vi "check syntax_core.vi"(8 "error in (no error)":errorcluster caption="에러 입력(에러 없음)", 11 "Script Line_i2c sw 입력":refnum<class "Script Line_i2c sw.lvclass">) -> (0 "error out":errorcluster caption="에러 출력", 3 "Script Line_i2c sw 출력":refnum<class "Script Line_i2c sw.lvclass">)   [LabVIEW 2020, in "Script Line_i2c sw.lvclass"]
uses:
  Script Line_i2c sw.lvclass
  Script Line/Script Line.lvclass/Script Line.ctl
  Script Line_i2c/Script Line_i2c.lvclass/Script Line_i2c.ctl
  Script Line_i2c/Accessors/Write slv.vi
  Script Line_i2c/Accessors/Write reg.vi
  Script Line_i2c/Accessors/Write reg addr byte.vi
  Script Line_i2c/Accessors/Write size.vi
  Script Line_i2c/Accessors/Write data.vi
  Script Line/Accessors/Read parameter.vi
  Script Line/Accessors/Read parameter string index.vi
  Script Line/Script Line.lvclass
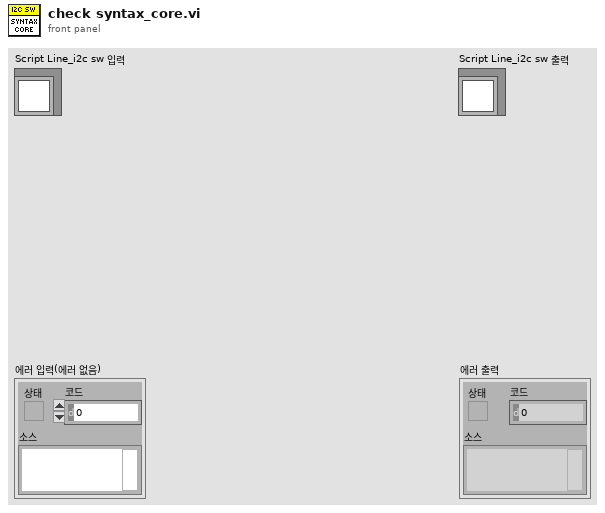
[diagram p1: front panel]
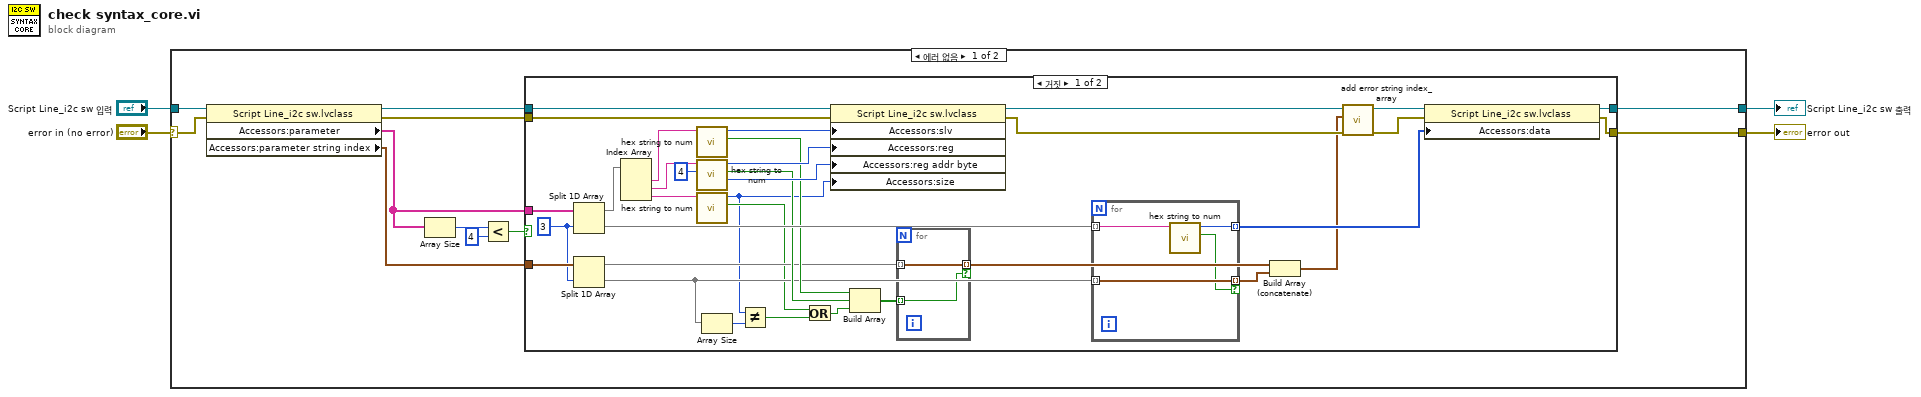
[diagram p0: block diagram]
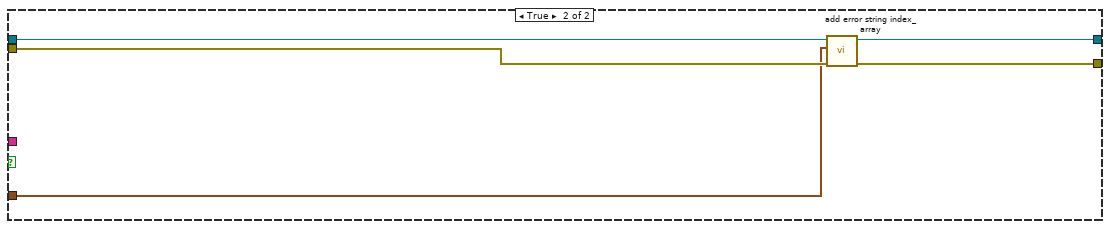
[diagram p2: hidden frame]
diagram:
  n1 = case shown="에러 없음" "error in (no error)" {
    selector: "error in (no error)" -> [w14 w62]
    tunnel: [w5 w62] -> w1
    tunnel: [w6 w61] -> w3
    tunnel: "Script Line_i2c sw 입력" -> [w15 w61]
    frame No Error {
      n2 = property class="Script Line_i2c sw.lvclass"(reference=w15, error in=w14) -> (reference out=w9:refnum<class "Script Line_i2c sw.lvclass">, error out=w8:errorcluster, "Accessors:parameter"=w10:string[], "Accessors:parameter string index"=w7:cluster{"start":u32, "end":u32}[])
      n3 = Array Size(array=w10) -> (size(s)=w13:i32)
      n4 = Less?(x=w13, y=4) -> (x < y?=w11:bool)
      n5 = case shown="거짓" w11 {
        tunnel: w10 -> [w49 _]
        tunnel: w7 -> [w48 w56]
        tunnel: w9 -> [w41 w58]
        tunnel: w8 -> [w42 w60]
        tunnel: [w45 w59] -> w5
        tunnel: [w43 w57] -> w6
        frame False {
          w37 = 3 ("길이")
          n6 = Split 1D Array(array=w49, index=w37) -> (first subarray=w36:string[], second subarray=w35:string[])
          n7 = Split 1D Array(array=w48, index=w37) -> (first subarray=w25:cluster{"start":u32, "end":u32}[], second subarray=w21:cluster{"start":u32, "end":u32}[])
          n8 = Index Array(array=w36) -> (element #1=w29:string, element #2=w30:string, element #3=w31:string)  [unwired: 3 in]
          n9 = call "hex string to num.vi"("string"=w29) -> ("error"=w27:bool, "num"=w32:u32)  [unwired: 7 in, 2 out]
          n10 = call "hex string to num.vi"("max byte (1)"=u8 4, "string"=w30) -> ("byte"=w39:u8, "error"=w26:bool, "num"=w40:u32)  [unwired: 6 in, 1 out]
          n11 = call "hex string to num.vi"("string"=w31) -> ("error"=w19:bool, "num"=w18:u32)  [unwired: 7 in, 2 out]
          n12 = Array Size(array=w21) -> (size(s)=w20:i32)
          n13 = Not Equal?(x=w18, y=w20) -> (x != y?=w16:bool)
          n14 = Or(x=w19, y=w16) -> (x .or. y?=w17:bool)
          n15 = property class="Script Line_i2c sw.lvclass"(reference=w41, error in=w42, "Accessors:slv"=w32, "Accessors:reg"=w40, "Accessors:reg addr byte"=w39, "Accessors:size"=w18) -> (reference out=w34:refnum<class "Script Line_i2c sw.lvclass">, error out=w33:errorcluster)
          n16 = Build Array(w27, w26, w17) -> (w24:bool[])
          n17 = for {
            tunnel: w25 -> [w51] mode=indexing
            tunnel: [w51] -> w22 mode=indexing if=w50
            tunnel: w24 -> [w50] mode=indexing
          }
          n18 = for {
            tunnel: w35 -> [w55] mode=indexing
            tunnel: w21 -> [w53] mode=indexing
            tunnel: [w54] -> w38 mode=indexing
            tunnel: [w53] -> w46 mode=indexing if=w52
            n19 = call "hex string to num.vi"("string"=w55) -> ("error"=w52:bool, "num"=w54:u32)  [unwired: 7 in, 2 out]
          }
          n20 = Build Array (concatenate)(w22, w46) -> (w23:cluster{"start":u32, "end":u32}[])
          n21 = call "add error string index_array.vi"("error in (no error)"=w33, "index_array"=w23, "Script Line 입력"=w34) -> ("error out"=w47:errorcluster, "Script Line 출력"=w44:refnum<class "Script Line_i2c sw.lvclass">)  [unwired: 7 in]
          n22 = property class="Script Line_i2c sw.lvclass"(reference=w44, error in=w47, "Accessors:data"=w38) -> (reference out=w43:refnum<class "Script Line_i2c sw.lvclass">, error out=w45:errorcluster)
        }
        frame True {
          n23 = call "add error string index_array.vi"("error in (no error)"=w60, "index_array"=w56, "Script Line 입력"=w58) -> ("error out"=w59:errorcluster, "Script Line 출력"=w57:refnum<class "Script Line_i2c sw.lvclass">)  [unwired: 7 in]
        }
      }
    }
    frame Error {
    }
  }
  "error out" <- w1
  "Script Line_i2c sw 출력" <- w3
